vi "hse-application_GetVersionInfos.vi"(8 "error in":errorcluster) -> (0 "error out":errorcluster, 1 "HSE-LIB Version":string, 2 "Framework Version":string, 3 "Application Version":string, 5 "FPGA Version":string, 7 "RT-App Version":string)   [LabVIEW 2014, in "hse-application.lvclass"]
doc: "Returns the various stored version numbers:\nApplication Version: This project (the built application)\nFramework Version: The HSE UI-Framework (Windows Application Template)\nHSE-LIB Version: The hse-libraries"
uses:
  hse-application.lvclass
  hse-application.lvclass/hse-application.ctl
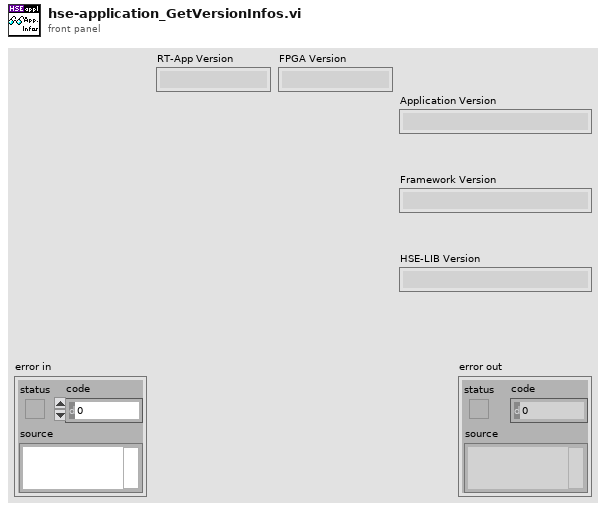
[diagram p1: front panel]
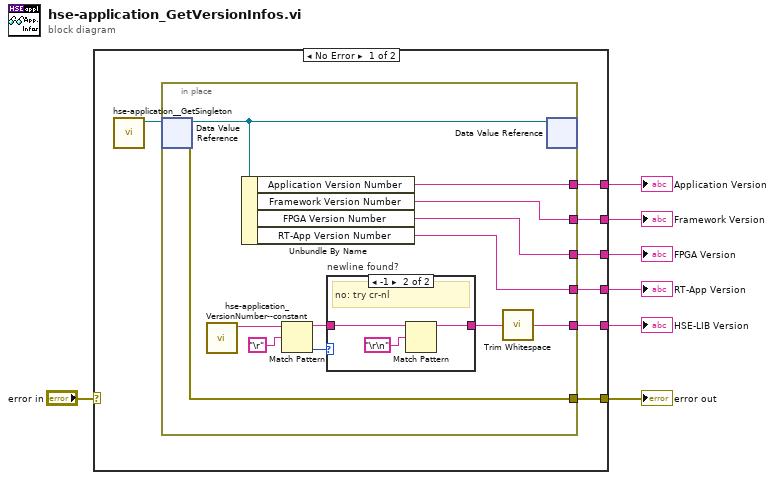
[diagram p0: block diagram]
diagram:
  n1 = case shown="No Error" "error in" {
    selector: "error in" -> [_ w31]
    tunnel: [w12 w31] -> w6
    tunnel: [w14 _] -> w3
    tunnel: [w11 _] -> w4
    tunnel: [w10 _] -> w5
    tunnel: [w9 _] -> w2
    tunnel: [w8 _] -> w1
    frame No Error {
      n2 = call "hse-application__GetSingleton.vi"() -> ("ApplicationClass DVR"=w13:refnum<data-value>)  [unwired: 10 in, 1 out]
      n3 = in-place {
        in-place-border: [w26] -> w14
        in-place-border: [w24] -> w12
        in-place-border: [w23] -> w11
        in-place-border: [w22] -> w10
        in-place-border: [w21] -> w9
        in-place-border: [w19] -> w8
        n4 = in-place-dvr #1(w13) -> (w25:refnum<class "hse-application.lvclass">, w24:errorcluster)
        n5 = call "hse-application_VersionNumber--constant.vi"() -> ("HSE-Libraries Version Number"=w15:string)  [unwired: 11 in]
        n6 = Unbundle By Name(w25) -> ("Application Version Number"=w22:string, "Framework Version Number"=w23:string, "FPGA Version Number"=w26:string, "RT-App Version Number"=w19:string)
        n7 = Match Pattern(string=w15, regular expression="\r") -> (before substring=w17:string, offset past match=w18:i32)  [unwired: 1 in, 2 out]
        n8 = case "newline found?" shown="-1" w18 {
          tunnel: w17 -> [w27 w29]
          tunnel: [w27 w28] -> w16
          frame Default {
            # "yes: do nothing"
          }
          frame -1 {
            # "no: try cr-nl"
            n9 = Match Pattern(string=w29, regular expression="\r\n") -> (before substring=w28:string)  [unwired: 1 in, 3 out]
          }
        }
        n10 = call <vilib>:"Trim Whitespace.vi"("string"=w16) -> ("trimmed string"=w21:string)  [unwired: 1 in]
        n11 = in-place-dvr #1(w25) -> ()  [unwired: 2 out]
      }
    }
    frame Error {
    }
  }
  "error out" <- w6
  "Application Version" <- w5
  "Framework Version" <- w4
  "FPGA Version" <- w3
  "HSE-LIB Version" <- w2
  "RT-App Version" <- w1
